vi "visualize.vi"() -> (3 "3D Picture 3":refnum<vi>(3d-picture), 10 "small angle":sgl, 11 "large axis angle":sgl)   [LabVIEW 2019]
uses:
  <vilib>/picture/3D Picture Control/Object/Create Object (name).vi
  <vilib>/picture/3D Picture Control/NI_3D Picture Control.lvlib
panel:
  out "error out":errorcluster
  in  "error in (no error)":errorcluster
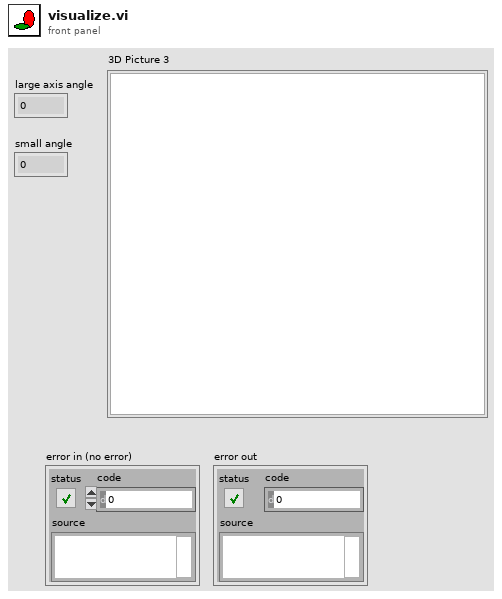
[diagram p1: front panel]
types:
  T1 = cluster{"Red":sgl, "Green":sgl, "Blue":sgl, "Alpha":sgl}
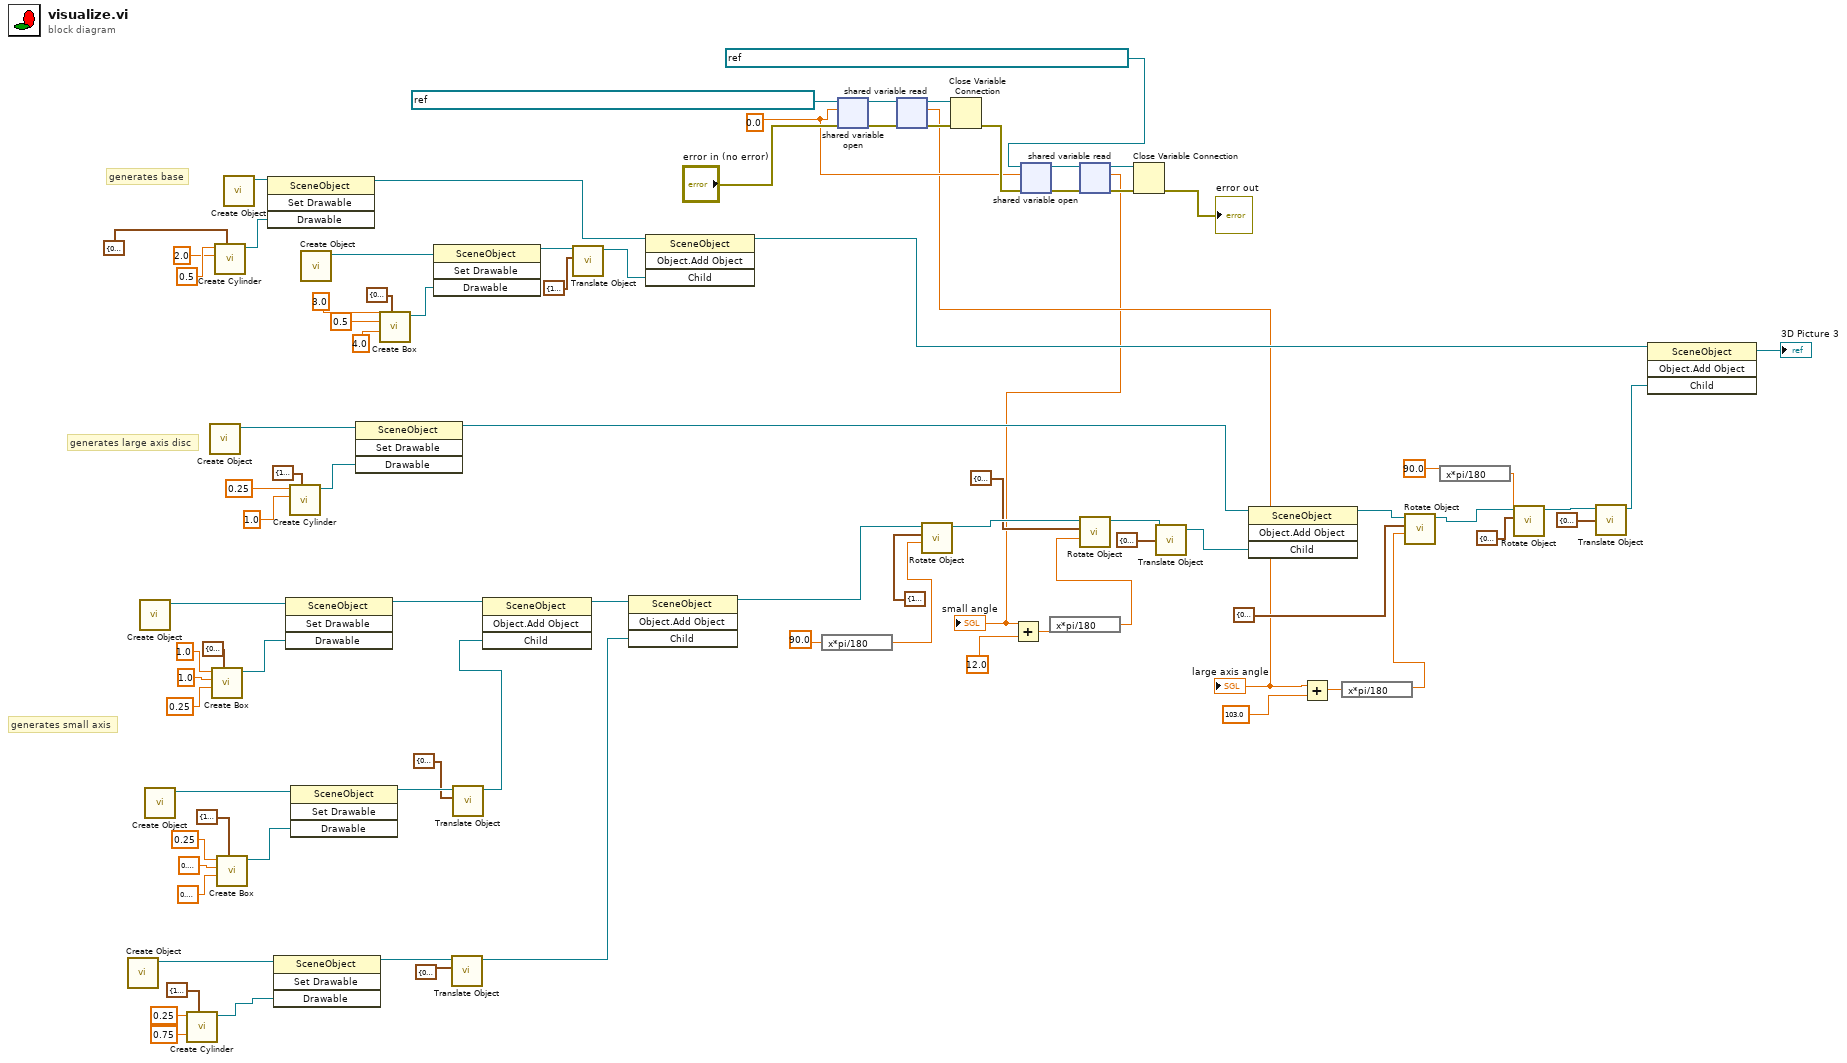
[diagram p0: block diagram]
diagram:
  w6 = sgl 0.0 ("Angle")
  # "generates small axis"
  # "generates large axis disc"
  # "generates base"
  n1 = call-poly <vilib>:"Create Object.vi"() -> ("Scene:New Object"=w75:refnum<vi>)  [unwired: 10 in, 1 out]
  n2 = call-poly <vilib>:"Create Object.vi"() -> ("Scene:New Object"=w88:refnum<vi>)  [unwired: 10 in, 1 out]
  n3 = call-poly <vilib>:"Create Object.vi"() -> ("Scene:New Object"=w77:refnum<vi>)  [unwired: 10 in, 1 out]
  n4 = call <vilib>:"Create Cylinder.vi"("Color"=T1 {"Red"=1.0, "Green"=1.0, "Blue"=1.0, "Alpha"=1.0}, "Radius"=sgl 0.75, "Height"=sgl 0.25) -> ("New Cylinder Refnum"=w74:refnum<vi>)  [unwired: 7 in, 1 out]
  n5 = call-poly <vilib>:"Create Object.vi"() -> ("Scene:New Object"=w60:refnum<vi>)  [unwired: 10 in, 1 out]
  n6 = call <vilib>:"Create Box.vi"("Color"=T1 {"Red"=0.0, "Green"=1.0, "Blue"=0.0, "Alpha"=1.0}, "Length Z"=sgl 0.25, "Length Y"=sgl 1.0, "Length X"=sgl 1.0) -> ("New Box Refnum"=w84:refnum<vi>)  [unwired: 6 in, 1 out]
  n7 = call <vilib>:"Create Cylinder.vi"("Color"=T1 {"Red"=0.8, "Green"=0.5, "Blue"=0.2, "Alpha"=1.0}, "Radius"=sgl 2.0, "Height"=sgl 0.5) -> ("New Cylinder Refnum"=w45:refnum<vi>)  [unwired: 7 in, 1 out]
  n8 = call <vilib>:"Create Box.vi"("Color"=T1 {"Red"=1.0, "Green"=1.0, "Blue"=0.0, "Alpha"=1.0}, "Length Z"=sgl 0.1, "Length Y"=sgl 0.1, "Length X"=sgl 0.25) -> ("New Box Refnum"=w81:refnum<vi>)  [unwired: 6 in, 1 out]
  n9 = call-poly <vilib>:"Create Object.vi"() -> ("Scene:New Object"=w44:refnum<vi>)  [unwired: 10 in, 1 out]
  n10 = invoke class="SceneObject" method="Set Drawable"(reference=w44, "Drawable"=w45) -> (reference out=w34:refnum<vi>)  [unwired: 2 in, 3 out]
  n11 = invoke class="SceneObject" method="Set Drawable"(reference=w75, "Drawable"=w74) -> (reference out=w69:refnum<vi>)  [unwired: 2 in, 3 out]
  n12 = invoke class="SceneObject" method="Set Drawable"(reference=w88, "Drawable"=w84) -> (reference out=w76:refnum<vi>)  [unwired: 2 in, 3 out]
  n13 = call <vilib>:"Create Cylinder.vi"("Color"=T1 {"Red"=1.0, "Green"=1.0, "Blue"=1.0, "Alpha"=1.0}, "Radius"=sgl 1.0, "Height"=sgl 0.25 ("Length Z")) -> ("New Cylinder Refnum"=w58:refnum<vi>)  [unwired: 7 in, 1 out]
  n14 = invoke class="SceneObject" method="Set Drawable"(reference=w77, "Drawable"=w81) -> (reference out=w66:refnum<vi>)  [unwired: 2 in, 3 out]
  n15 = call-poly <vilib>:"Create Object.vi"() -> ("Scene:New Object"=w43:refnum<vi>)  [unwired: 10 in, 1 out]
  n16 = invoke class="SceneObject" method="Set Drawable"(reference=w60, "Drawable"=w58) -> (reference out=w55:refnum<vi>)  [unwired: 2 in, 3 out]
  n17 = call <vilib>:"Create Box.vi"("Color"=T1 {"Red"=0.8, "Green"=0.5, "Blue"=0.2, "Alpha"=1.0}, "Length Z"=sgl 4.0, "Length Y"=sgl 3.0, "Length X"=sgl 0.5) -> ("New Box Refnum"=w40:refnum<vi>)  [unwired: 6 in, 1 out]
  n18 = invoke class="SceneObject" method="Set Drawable"(reference=w43, "Drawable"=w40) -> (reference out=w36:refnum<vi>)  [unwired: 2 in, 3 out]
  n19 = call <vilib>:"Translate Object.vi"("Translation"=cluster{"X":sgl, "Y":sgl, "Z":sgl} {"X"=0.0, "Y"=0.0, "Z"=-0.25}, "Scene.Object In"=w69) -> ("Scene.Object Out"=w67:refnum<vi>)  [unwired: 8 in, 1 out]
  n20 = call <vilib>:"Translate Object.vi"("Translation"=cluster{"X":sgl, "Y":sgl, "Z":sgl} {"X"=0.4, "Y"=0.0, "Z"=0.1}, "Scene.Object In"=w66) -> ("Scene.Object Out"=w64:refnum<vi>)  [unwired: 8 in, 1 out]
  n21 = invoke class="SceneObject" method="Object.Add Object"(reference=w76, "Child"=w64) -> (reference out=w70:refnum<vi>)  [unwired: 2 in, 3 out]
  n22 = call <vilib>:"Translate Object.vi"("Translation"=cluster{"X":sgl, "Y":sgl, "Z":sgl} {"X"=1.0, "Y"=0.0, "Z"=2.0}, "Scene.Object In"=w36) -> ("Scene.Object Out"=w35:refnum<vi>)  [unwired: 8 in, 1 out]
  n23 = invoke class="SceneObject" method="Object.Add Object"(reference=w70, "Child"=w67) -> (reference out=w50:refnum<vi>)  [unwired: 2 in, 3 out]
  n24 = invoke class="SceneObject" method="Object.Add Object"(reference=w34, "Child"=w35) -> (reference out=w32:refnum<vi>)  [unwired: 2 in, 3 out]
  n25 = expression code="x*pi/180"(sgl 90.0 ("small axis angle")) -> (w61:sgl)
  n26 = shared-variable-open(refnum<k21> "ni.var.psp://housesoftheholy/Attocube 3DR/axis 1%3A current position" ("shared variable refnum in"), "error in (no error)", w6) -> (w16:refnum<k21>, w15:errorcluster)  [unwired: 1 in]
  n27 = shared-variable-read(w16, w15) -> (w4:refnum<k21>, w14:errorcluster, w5:sgl)  [unwired: 1 out]
  "large axis angle" <- w5
  n28 = call <vilib>:"Rotate Object.vi"("Angle"=w61, "Axis"=cluster{"X":sgl, "Y":sgl, "Z":sgl} {"X"=1.0, "Y"=0.0, "Z"=0.0} ("rotate small axis"), "Scene.Object In"=w50) -> ("Scene.Object Out"=w52:refnum<vi>)  [unwired: 7 in, 1 out]
  n29 = Close Variable Connection(8:w14, 11:w4) -> (0:w9:errorcluster)
  n30 = shared-variable-open(refnum<k21> "ni.var.psp://housesoftheholy/Attocube 3DR/axis 2%3A current position" ("shared variable refnum in"), w9, w6) -> (w10:refnum<k21>, w11:errorcluster)  [unwired: 1 in]
  n31 = shared-variable-read(w10, w11) -> (w3:refnum<k21>, w12:errorcluster, w2:sgl)  [unwired: 1 out]
  "small angle" <- w2
  n32 = Add(x=w2, y=sgl 12.0 ("y 2")) -> (x+y=w20:sgl)
  n33 = expression code="x*pi/180"(w20) -> (w19:sgl)
  n34 = call <vilib>:"Rotate Object.vi"("Angle"=w19, "Axis"=cluster{"X":sgl, "Y":sgl, "Z":sgl} {"X"=0.0, "Y"=1.0, "Z"=0.0} ("small axis"), "Scene.Object In"=w52) -> ("Scene.Object Out"=w49:refnum<vi>)  [unwired: 7 in, 1 out]
  n35 = Close Variable Connection(8:w12, 11:w3) -> (0:→"error out":errorcluster)
  n36 = call <vilib>:"Translate Object.vi"("Translation"=cluster{"X":sgl, "Y":sgl, "Z":sgl} {"X"=0.0, "Y"=0.5, "Z"=-1.0} ("translate small axis"), "Scene.Object In"=w49) -> ("Scene.Object Out"=w47:refnum<vi>)  [unwired: 8 in, 1 out]
  n37 = invoke class="SceneObject" method="Object.Add Object"(reference=w55, "Child"=w47) -> (reference out=w54:refnum<vi>)  [unwired: 2 in, 3 out]
  n38 = Add(x=w5, y=sgl 103.0) -> (x+y=w18:sgl)
  n39 = expression code="x*pi/180"(w18) -> (w17:sgl)
  n40 = call <vilib>:"Rotate Object.vi"("Angle"=w17, "Axis"=cluster{"X":sgl, "Y":sgl, "Z":sgl} {"X"=0.0, "Y"=0.0, "Z"=1.0} ("Large axis"), "Scene.Object In"=w54) -> ("Scene.Object Out"=w30:refnum<vi>)  [unwired: 7 in, 1 out]
  n41 = expression code="x*pi/180"(sgl 90.0 ("Angle")) -> (w24:sgl)
  n42 = call <vilib>:"Rotate Object.vi"("Angle"=w24, "Axis"=cluster{"X":sgl, "Y":sgl, "Z":sgl} {"X"=0.0, "Y"=1.0, "Z"=0.0}, "Scene.Object In"=w30) -> ("Scene.Object Out"=w29:refnum<vi>)  [unwired: 7 in, 1 out]
  n43 = call <vilib>:"Translate Object.vi"("Translation"=cluster{"X":sgl, "Y":sgl, "Z":sgl} {"X"=0.5, "Y"=0.0, "Z"=3.0}, "Scene.Object In"=w29) -> ("Scene.Object Out"=w28:refnum<vi>)  [unwired: 8 in, 1 out]
  n44 = invoke class="SceneObject" method="Object.Add Object"(reference=w32, "Child"=w28) -> (reference out=→"3D Picture 3":refnum<vi>)  [unwired: 2 in, 3 out]
